vi "Absolute Accuracy ZYLCRXGB.vi"(8 "error in (no error)":errorcluster, 9 "Acal":dbl format="%.2f", 10 "Ae":dbl format="%.2f", 11 "VISA resource name":refnum<visa-resource-name>) -> (0 "error out":errorcluster, 2 "Absolute Accuracy":dbl format="%.2f", 3 "VISA resource name out":refnum<visa-resource-name>)   [LabVIEW 2015, in "Agilent 428X Series.lvlib"]
doc: "ThisVI calculates the absolute accuracy for Z, Y, L, C, R, X, G, and B accuracy (Given as Ae+Aca).\n\nNote: L, C, X, B accuracies apply when Dx <=0.1.\n R and G apply only when Qx<=0.1.\n G accuracy is only valid under G-B combination measurement.\n\nDisclaimer: All accuracy calculation VI's are not part of the original \n driver. They are provided for supplementry purpose only.\n If user desires very high accuracy data, please do or \n check the calculation seperately."
uses:
  <instrlib>/Agilent 428X Series/Agilent 428X Series.lvlib
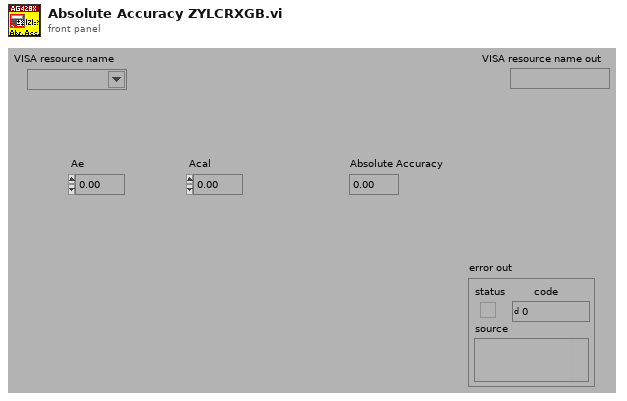
[diagram p1: front panel]
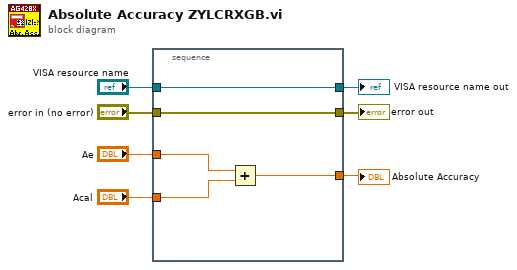
[diagram p0: block diagram]
diagram:
  n1 = stacked-sequence {
    tunnel: "Ae" -> [w12]
    tunnel: "Acal" -> [w11]
    tunnel: [w10] -> w5
    tunnel: "VISA resource name" -> [w9]
    tunnel: [w9] -> w3
    tunnel: "error in (no error)" -> [w8]
    tunnel: [w8] -> w1
    frame #0 {
      n2 = Add(x=w12, y=w11) -> (x+y=w10:dbl)
    }
  }
  "VISA resource name out" <- w3
  "error out" <- w1
  "Absolute Accuracy" <- w5
